vi "RSLATCH.vi"(5 "Reset":bool, 11 "Set":bool) -> (3 "Output":bool)   [LabVIEW 2015]
doc: "When S is given an input of true, this VI will be set on; it will stay true as long as it is set. The VI resets when the R input turns on; it will then return false and wait for S to turn on again.\n\nIf both inputs are true, the Reset is given priority and the input is set to false."
uses:
  <vilib>/functionblocks/Bistables/RS Bistable/RS Bistable.vi
  <vilib>/functionblocks/FB Core/FB Core.xnode
  <vilib>/functionblocks/NI_FunctionBlock Libraries.lvlib
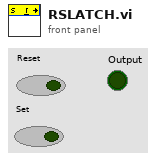
[diagram p1: front panel]
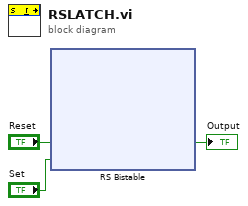
[diagram p0: block diagram]
diagram:
  n1 = xnode "RS Bistable"("reset"="Reset", "set"="Set") -> ("output"=→"Output":bool)  [unwired: 1 in, 1 out]
